vi "Sets the SCPI Mode.vi"(5 "Enable to Query":bool=TRUE, 7 "Enable to Sets":bool=TRUE, 8 "error in":errorcluster, 10 "SCPI Mode":u16(ring) items=["Normal", "Compatible"], 11 "VISA resource name":refnum<visa-resource-name>) -> (0 "error out":errorcluster, 2 "Returns the SCPI Mode":string, 3 "VISA resource name out":refnum<visa-resource-name>)   [LabVIEW 2011, in "DMM4.lvlib"]
uses:
  <instrlib>/DMM4/DMM4.lvlib
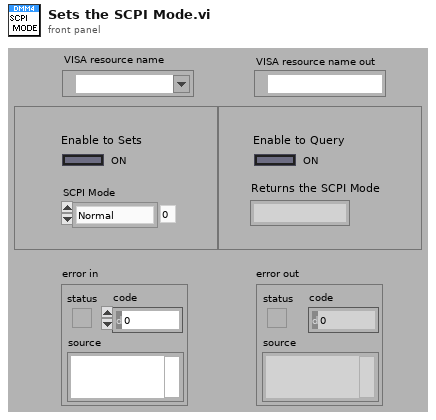
[diagram p1: front panel]
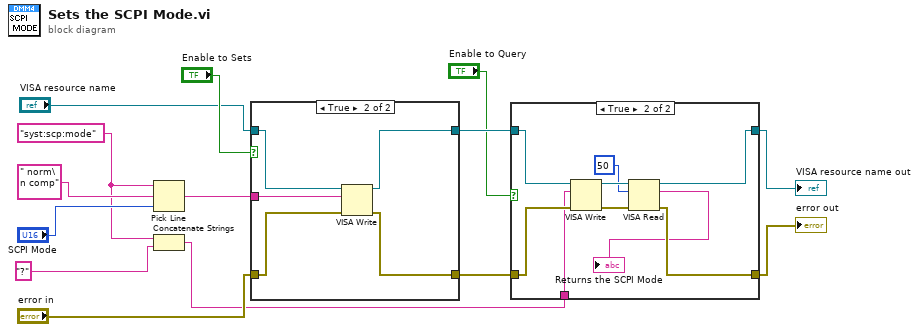
[diagram p0: block diagram]
diagram:
  w11 = "syst:scp:mode"
  n1 = Pick Line(string ("")=w11, multi-line string=" norm\n comp", line index="SCPI Mode") -> (output string=w7:string)
  n2 = Concatenate Strings(w11, "?") -> (w4:string)
  n3 = case shown="True" "Enable to Sets" {
    tunnel: "VISA resource name" -> [w16 w21]
    tunnel: "error in" -> [w15 w20]
    tunnel: [w16 w19] -> w6
    tunnel: [w15 w18] -> w5
    tunnel: w7 -> [_ w17]
    frame False {
    }
    frame True {
      n4 = VISA Write(VISA resource name=w21, write buffer=w17, error in (no error)=w20) -> (VISA resource name out=w19:refnum<visa-resource-name>, error out=w18:errorcluster)  [unwired: 1 out]
    }
  }
  n5 = case shown="True" "Enable to Query" {
    tunnel: w6 -> [w23 w30]
    tunnel: [w23 w28] -> w2
    tunnel: w5 -> [w22 w29]
    tunnel: [w22 w27] -> w1
    tunnel: w4 -> [_ w25]
    frame False {
    }
    frame True {
      n6 = VISA Write(VISA resource name=w30, write buffer=w25, error in (no error)=w29) -> (VISA resource name out=w31:refnum<visa-resource-name>, error out=w32:errorcluster)  [unwired: 1 out]
      n7 = VISA Read(VISA resource name=w31, byte count=u32 50, error in (no error)=w32) -> (VISA resource name out=w28:refnum<visa-resource-name>, read buffer=→"Returns the SCPI Mode":string, error out=w27:errorcluster)  [unwired: 1 out]
    }
  }
  "VISA resource name out" <- w2
  "error out" <- w1
